vi "AlliGator Update Phasor References v2.vi"(0 "XYGraph in":refnum<vi>, 1 "Phasor Frequency":dbl[unit]=160000000.0, 5 "Phase Lifetime 1":refnum<vi>, 7 "Phase Lifetime 2":refnum<vi>, 9 "New Reference Phase":dbl, 11 "Error In":errorcluster, 12 "Locked Plots":i32[](array[numeric]), 13 "Updated Reference ID":i32) -> (4 "Reference Phasor 1":T1, 6 "Reference Lifetime 1":dbl[unit], 8 "Reference Phasor 2":T1, 10 "Reference Lifetime 2":dbl[unit], 15 "Error Out":errorcluster)   [LabVIEW 2021, in "AlliGator Phasor Graph.lvlib"]
doc: "Updates phasor references using the internally stored information.\n\nGenerally, this happens after the phasor harmonic has been changed."
uses:
  AlliGator Phasor Graph.lvlib
  Phasor/Phasor (g, s).ctl
  Phasor/Phasor.lvlib
panel:
  in  "Move Both References?":bool=TRUE
  # "see the AlliGator License on the block diagram (Ctrl+E or Window:Show Block Diagram)"
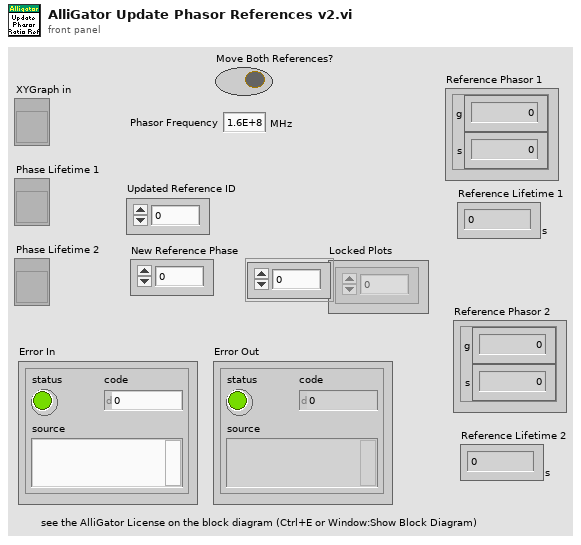
[diagram p1: front panel]
types:
  T1 = typedef "Phasor.lvlib/Phasor (g, s).ctl" = cluster{"g":dbl, "s":dbl}
  T2 = typedef "LVAnnotationListTypeDef.ctl" = cluster{"Name":string, "Color":u32, "Style":u8, "Point Style":u8, "Name Visible":bool, "Allow Drag":bool, "Annotation Mode":u32, "Plot":i32, "Index":i32, "Position":cluster{"X":dbl, "Y":dbl}, "X Scale":u32, "Y Scale":u32, "Show Arrow":bool, "Lock Name":bool, "Plot Area":i32, "Label Offset":cluster{"X":dbl, "Y":dbl}}[]
  T3 = typedef "LVCursorListTypeDef.ctl" = cluster{"Name":string, "Color":u32, "Style":u8, "Point Style":u8, "Name Visible":bool, "Allow Drag":bool, "Cursor Mode":u32, "Plot":i32, "Index":i32, "Position":cluster{"X":dbl, "Y":dbl}, "X Scale":u32, "Y Scale":u32, "Watch Plots":i32[], "Watch All Plots":bool, "Plot Area":i32, "Label Offset":cluster{"X":dbl, "Y":dbl}}[]
  T4 = typedef "Phasor.lvlib/Phasor (m, phi).ctl" = cluster{"m":dbl, "phi":dbl}
  T5 = cluster{"Name":string, "Color":u32, "Style":u8, "Point Style":u8, "Name Visible":bool, "Allow Drag":bool, "Annotation Mode":u32, "Plot":i32, "Index":i32, "Position":cluster{"X":dbl, "Y":dbl}, "X Scale":u32, "Y Scale":u32, "Show Arrow":bool, "Lock Name":bool, "Plot Area":i32, "Label Offset":cluster{"X":dbl, "Y":dbl}}
  T6 = cluster{"Name":string, "Color":u32, "Style":u8, "Point Style":u8, "Name Visible":bool, "Allow Drag":bool, "Cursor Mode":u32, "Plot":i32, "Index":i32, "Position":cluster{"X":dbl, "Y":dbl}, "X Scale":u32, "Y Scale":u32, "Watch Plots":i32[], "Watch All Plots":bool, "Plot Area":i32, "Label Offset":cluster{"X":dbl, "Y":dbl}}
  T7 = cluster{"Numeric Control":dbl, "Numeric Control":dbl}
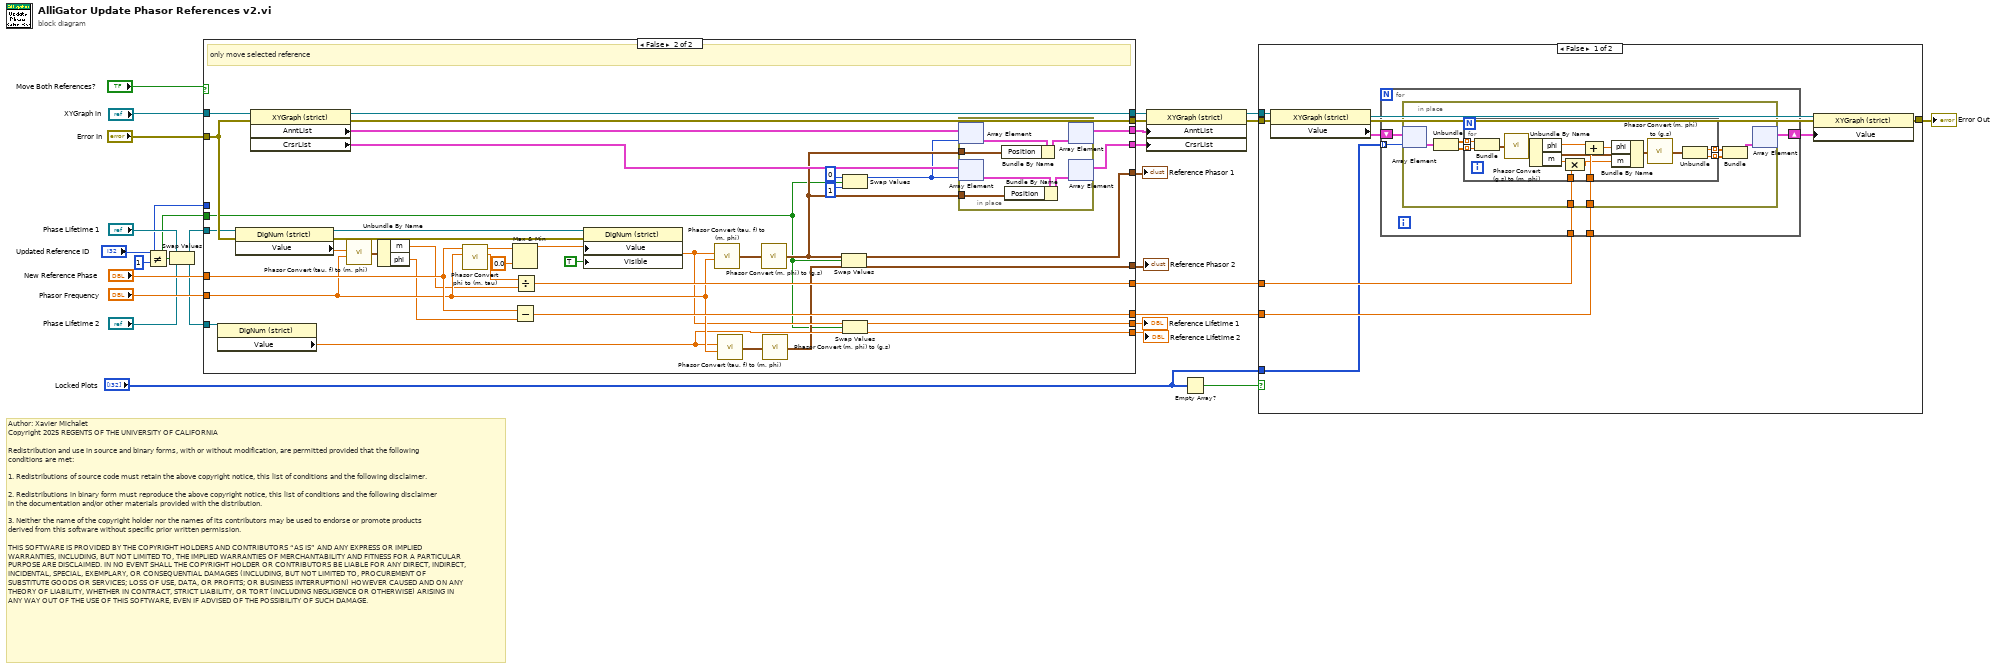
[diagram p0: block diagram]
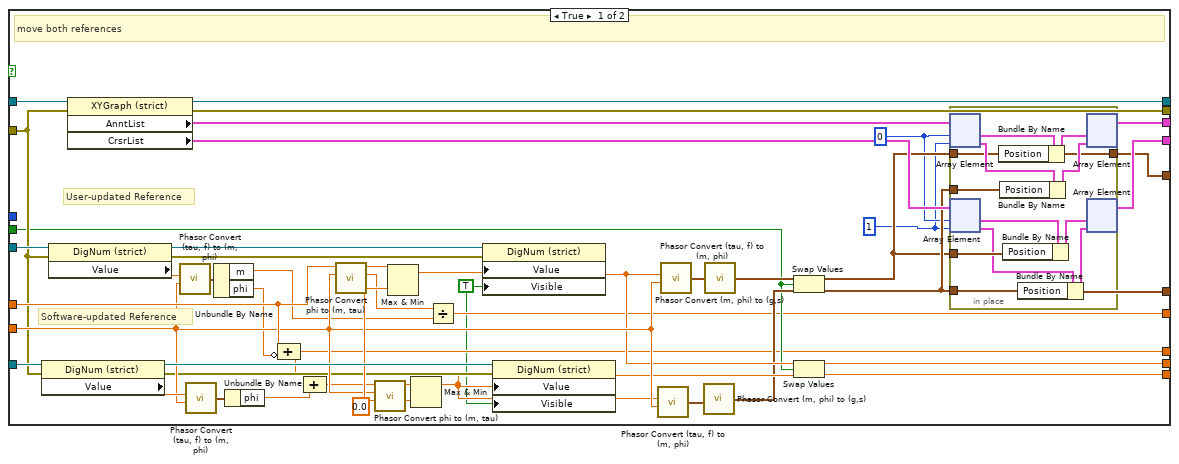
[diagram p2: hidden frame]
diagram:
  # "Author: Xavier Michalet\nCopyright 2025 REGENTS OF THE UNIVERSITY OF CALIFORNIA\n\nRedistribution and use in source and binary forms, with or without modification, are permitted provided that the following conditions are met:\n\n1. Redistributions of source code must retain the above copyright notice, this list of conditions and the following disclaimer.\n\n2. Redistributions in binary form must reproduce the above copyright notice, this list of conditions and the following disclaimer in the documentation and/or other materials provided with the distribution.\n\n3. Neither the name of the copyright holder nor the names of its contributors may be used to endorse or promote products derived from this software without specific prior written permission.\n\nTHIS SOFTWARE IS PROVIDED BY THE COPYRIGHT HOLDERS AND CONTRIBUTORS “AS IS” AND ANY EXPRESS OR IMPLIED WARRANTIES, INCLUDING, BUT NOT LIMITED TO, THE IMPLIED WARRANTIES OF MERCHANTABILITY AND FITNESS FOR A PARTICULAR PURPOSE ARE DISCLAIMED. IN NO EVENT SHALL THE COPYRIGHT HOLDER OR CONTRIBUTORS BE LIABLE FOR ANY DIRECT, INDIRECT, INCIDENTAL, SPECIAL, EXEMPLARY, OR CONSEQUENTIAL DAMAGES (INCLUDING, BUT NOT LIMITED TO, PROCUREMENT OF SUBSTITUTE GOODS OR SERVICES; LOSS OF USE, DATA, OR PROFITS; OR BUSINESS INTERRUPTION) HOWEVER CAUSED AND ON ANY THEORY OF LIABILITY, WHETHER IN CONTRACT, STRICT LIABILITY, OR TORT (INCLUDING NEGLIGENCE OR OTHERWISE) ARISING IN ANY WAY OUT OF THE USE OF THIS SOFTWARE, EVEN IF ADVISED OF THE POSSIBILITY OF SUCH DAMAGE."
  n1 = Not Equal?(x="Updated Reference ID", y=1) -> (x != y?=w1:bool)
  n2 = Swap Values(12:"Phase Lifetime 1", 13:w1, 14:"Phase Lifetime 2") -> (1:w6:refnum<vi>, 3:w5:refnum<vi>)
  n3 = case shown="False" "Move Both References?" {
    tunnel: "XYGraph in" -> [w72 w122]
    tunnel: w5 -> [w71 w102]
    tunnel: w6 -> [w69 w103]
    tunnel: "New Reference Phase" -> [w65 w110]
    tunnel: "Phasor Frequency" -> [w61 w104]
    tunnel: [w60 w118] -> w24
    tunnel: [w58 w116] -> w23
    tunnel: [w56 w114] -> w22
    tunnel: "Error In" -> [w55 w113]
    tunnel: [w52 w111] -> w20
    tunnel: [w34 w109] -> w15
    tunnel: [w35 w106] -> w14
    tunnel: [w43 w98] -> w12
    tunnel: [w44 w99] -> w13
    tunnel: [w47 w94] -> w11
    tunnel: [w40 w96] -> w10
    tunnel: "Updated Reference ID" -> [_ _]
    tunnel: w1 -> [w36 w93]
    frame True {
      w28 = TRUE ("Visible")
      w37 = 1
      w38 = 0
      w62 = dbl[unit] 0.0 ("y")
      # "Software-updated Reference"
      # "User-updated Reference"
      # "move both references"
      n4 = property class="DigNum (strict)"(reference=w71, error in=w55) -> (reference out=w70:refnum<vi>, error out=w53:errorcluster, "Value"=w67:dbl[unit])
      n5 = property class="DigNum (strict)"(reference=w69, error in=w55) -> (reference out=w68:refnum<vi>, error out=w54:errorcluster, "Value"=w66:dbl[unit])
      n6 = property class="XYGraph (strict)"(reference=w72, error in=w55) -> (reference out=w60:refnum<vi>, error out=w52:errorcluster, "AnntList"=w59:T2, "CrsrList"=w57:T3)
      n7 = call "Phasor Convert (tau, f) to (m, phi).vi"("Lifetime"=w66, "Phasor Frequency"=w61) -> ("Phasor (m, phi)"=w48:T4)  [unwired: 5 in]
      n8 = call "Phasor Convert (tau, f) to (m, phi).vi"("Lifetime"=w67, "Phasor Frequency"=w61) -> ("Phasor (m, phi)"=w51:T4)  [unwired: 5 in]
      n9 = Unbundle By Name(w48) -> ("m"=w31:dbl, "phi"=w30:dbl)
      n10 = Unbundle By Name(w51) -> ("phi"=w29:dbl)
      n11 = Compound Arithmetic op=ADD(w65, invert w30) -> (w34:dbl)
      n12 = Compound Arithmetic op=ADD(w34, w29) -> (w50:dbl)
      n13 = call "Phasor Convert phi to (m, tau).vi"("Phasor Frequency"=w61, "Phase"=w65) -> ("Modulus"=w49:dbl, "Phase Lifetime"=w63:dbl[unit])  [unwired: 8 in]
      n14 = call "Phasor Convert phi to (m, tau).vi"("Phasor Frequency"=w61, "Phase"=w50) -> ("Phase Lifetime"=w64:dbl[unit])  [unwired: 8 in, 1 out]
      n15 = Max & Min(x=w63, y=w62) -> (max(x,y)=w46:dbl[unit])  [unwired: 1 out]
      n16 = Max & Min(x=w64, y=w62) -> (max(x,y)=w45:dbl[unit])  [unwired: 1 out]
      n17 = Divide(x=w49, y=w31) -> (x/y=w35:dbl)
      n18 = property class="DigNum (strict)"(reference=w68, error in=w54, "Value"=w46, "Visible"=w28) -> ()  [unwired: 2 out]
      n19 = property class="DigNum (strict)"(reference=w70, error in=w53, "Value"=w45, "Visible"=w28) -> ()  [unwired: 2 out]
      n20 = call "Phasor Convert (tau, f) to (m, phi).vi"("Lifetime"=w45, "Phasor Frequency"=w61) -> ("Phasor (m, phi)"=w32:T4)  [unwired: 5 in]
      n21 = call "Phasor Convert (tau, f) to (m, phi).vi"("Lifetime"=w46, "Phasor Frequency"=w61) -> ("Phasor (m, phi)"=w33:T4)  [unwired: 5 in]
      n22 = call "Phasor Convert (m, phi) to (g,s).vi"("Phasor (m, phi)"=w32) -> ("Phasor (g, s)"=w41:T1)  [unwired: 8 in]
      n23 = call "Phasor Convert (m, phi) to (g,s).vi"("Phasor (m, phi)"=w33) -> ("Phasor (g, s)"=w42:T1)  [unwired: 8 in]
      n24 = Swap Values(12:w42, 13:w36, 14:w41) -> (1:w39:T1, 3:w40:T1)
      n25 = Swap Values(12:w46, 13:w36, 14:w45) -> (1:w44:dbl[unit], 3:w43:dbl[unit])
      n26 = in-place {
        in-place-border: w39 -> [w73]
        in-place-border: w40 -> [w82]
        in-place-border: w39 -> [w78]
        in-place-border: w40 -> [w74]
        in-place-border: [w73] -> w47
        n27 = in-place-array #1(w59, w38, w37) -> (w81:T5, w84:T5)
        n28 = in-place-array #2(w57, w38, w37) -> (w79:T6, w76:T6)
        n29 = Bundle By Name(cluster=w81, "Position"=w73) -> (w80:T5)
        n30 = Bundle By Name(cluster=w84, "Position"=w82) -> (w83:T5)
        n31 = Bundle By Name(cluster=w79, "Position"=w78) -> (w77:T6)
        n32 = Bundle By Name(cluster=w76, "Position"=w74) -> (w75:T6)
        n33 = in-place-array #1(w80, w83) -> (w58:T2)  [unwired: 2 out]
        n34 = in-place-array #2(w77, w75) -> (w56:T3)  [unwired: 2 out]
      }
    }
    frame False {
      # "only move selected reference"
      n35 = property class="DigNum (strict)"(reference=w102) -> ("Value"=w100:dbl[unit])  [unwired: 1 in, 2 out]
      n36 = property class="DigNum (strict)"(reference=w103, error in=w113) -> (reference out=w121:refnum<vi>, error out=w112:errorcluster, "Value"=w120:dbl[unit])
      n37 = property class="XYGraph (strict)"(reference=w122, error in=w113) -> (reference out=w118:refnum<vi>, error out=w111:errorcluster, "AnntList"=w117:T2, "CrsrList"=w115:T3)
      n38 = call "Phasor Convert (tau, f) to (m, phi).vi"("Lifetime"=w120, "Phasor Frequency"=w104) -> ("Phasor (m, phi)"=w107:T4)  [unwired: 5 in]
      n39 = Unbundle By Name(w107) -> ("m"=w87:dbl, "phi"=w86:dbl)
      n40 = call "Phasor Convert phi to (m, tau).vi"("Phasor Frequency"=w104, "Phase"=w110) -> ("Modulus"=w108:dbl, "Phase Lifetime"=w119:dbl[unit])  [unwired: 8 in]
      n41 = Max & Min(x=w119, y=dbl[unit] 0.0) -> (max(x,y)=w101:dbl[unit])  [unwired: 1 out]
      n42 = Subtract(x=w110, y=w86) -> (x-y=w109:dbl)
      n43 = Divide(x=w108, y=w87) -> (x/y=w106:dbl)
      n44 = property class="DigNum (strict)"(reference=w121, error in=w112, "Value"=w101, "Visible"=TRUE) -> ()  [unwired: 2 out]
      n45 = call "Phasor Convert (tau, f) to (m, phi).vi"("Lifetime"=w101, "Phasor Frequency"=w104) -> ("Phasor (m, phi)"=w89:T4)  [unwired: 5 in]
      n46 = call "Phasor Convert (tau, f) to (m, phi).vi"("Lifetime"=w100, "Phasor Frequency"=w104) -> ("Phasor (m, phi)"=w88:T4)  [unwired: 5 in]
      n47 = call "Phasor Convert (m, phi) to (g,s).vi"("Phasor (m, phi)"=w89) -> ("Phasor (g, s)"=w95:T1)  [unwired: 8 in]
      n48 = call "Phasor Convert (m, phi) to (g,s).vi"("Phasor (m, phi)"=w88) -> ("Phasor (g, s)"=w97:T1)  [unwired: 8 in]
      n49 = Swap Values(12:w95, 13:w93, 14:w97) -> (1:w94:T1, 3:w96:T1)
      n50 = Swap Values(12:0 ("y"), 13:w93, 14:1 ("x")) -> (1:w90:i32)  [unwired: 1 out]
      n51 = Swap Values(12:w101, 13:w93, 14:w100) -> (1:w99:dbl[unit], 3:w98:dbl[unit])
      n52 = in-place {
        in-place-border: w95 -> [w124]
        in-place-border: w95 -> [w123]
        n53 = in-place-array #3(w117, w90) -> (w128:T5)
        n54 = in-place-array #4(w115, w90) -> (w126:T6)
        n55 = Bundle By Name(cluster=w128, "Position"=w124) -> (w127:T5)
        n56 = Bundle By Name(cluster=w126, "Position"=w123) -> (w125:T6)
        n57 = in-place-array #3(w127) -> (w116:T2)  [unwired: 1 out]
        n58 = in-place-array #4(w125) -> (w114:T3)  [unwired: 1 out]
      }
    }
  }
  "Reference Lifetime 1" <- w13
  "Reference Lifetime 2" <- w12
  "Reference Phasor 1" <- w11
  "Reference Phasor 2" <- w10
  n59 = property class="XYGraph (strict)"(reference=w24, error in=w20, "AnntList"=w23, "CrsrList"=w22) -> (reference out=w19:refnum<vi>, error out=w18:errorcluster)
  n60 = Empty Array?(array="Locked Plots") -> (empty?=w9:bool)
  n61 = case shown="False" w9 {
    tunnel: w19 -> [w138 _]
    tunnel: w18 -> [w137 w166]
    tunnel: [w132 w166] -> w17
    tunnel: w15 -> [w131 _]
    tunnel: w14 -> [w130 _]
    tunnel: "Locked Plots" -> [w129 _]
    frame False {
      n62 = property class="XYGraph (strict)"(reference=w138, error in=w137) -> (reference out=w134:refnum<vi>, error out=w133:errorcluster, "Value"=w136:cluster{"X Array":dbl[], "Y Array":dbl[]}[])
      n63 = for {
        tunnel: w131 -> [w141]
        tunnel: w130 -> [w140]
        shift-right: [w142] -> w135
        shift-left: w136 -> [w143]
        tunnel: w129 -> [w139] mode=indexing
        n64 = in-place {
          in-place-border: w141 -> [w148]
          in-place-border: w140 -> [w147]
          n65 = in-place-array #5(w143, w139) -> (w151:cluster{"X Array":dbl[], "Y Array":dbl[]})
          n66 = Unbundle(w151) -> ("X Array"=w150:dbl[], "Y Array"=w149:dbl[])
          n67 = for {
            tunnel: w150 -> [w165] mode=indexing
            tunnel: w149 -> [w164] mode=indexing
            tunnel: w148 -> [w161]
            tunnel: w147 -> [w159]
            tunnel: [w153] -> w146 mode=indexing
            tunnel: [w152] -> w145 mode=indexing
            n68 = Bundle("Numeric Control"=w165, "Numeric Control"=w164) -> (w163:T7)  [unwired: 1 in]
            n69 = call "Phasor Convert (g,s) to (m, phi).vi"("Phasor (g, s)"=w163) -> ("Phasor (m, phi)"=w158:T4)  [unwired: 8 in]
            n70 = Unbundle By Name(w158) -> ("phi"=w162:dbl, "m"=w160:dbl)
            n71 = Compound Arithmetic op=MULTIPLY(w160, w159) -> (w156:dbl)
            n72 = Compound Arithmetic op=ADD(w162, w161) -> (w157:dbl)
            n73 = Bundle By Name(cluster=w158, "phi"=w157, "m"=w156) -> (w155:T4)
            n74 = call "Phasor Convert (m, phi) to (g,s).vi"("Phasor (m, phi)"=w155) -> ("Phasor (g, s)"=w154:T1)  [unwired: 8 in]
            n75 = Unbundle(w154) -> ("g"=w153:dbl, "s"=w152:dbl)
          }
          n76 = Bundle(w146, w145) -> (w144:cluster{dbl[], dbl[]})  [unwired: 1 in]
          n77 = in-place-array #5(w144) -> (w142:cluster{"X Array":dbl[], "Y Array":dbl[]}[])  [unwired: 1 out]
        }
      }
      n78 = property class="XYGraph (strict)"(reference=w134, error in=w133, "Value"=w135) -> (error out=w132:errorcluster)  [unwired: 1 out]
    }
    frame True {
      # "no plot locked"
    }
  }
  "Error Out" <- w17
